vi "SEQ Header Read.vi"(0 "refnum":refnum<file>, 11 "error in":errorcluster) -> (4 "refnum out":refnum<file>, 6 "# of Frames":i16, 8 "AOI List":i16[][](array[numeric]), 10 "Header Info":T1, 15 "error out":errorcluster)   [LabVIEW 2011]
panel:
  # "Reading Sequence File Header"
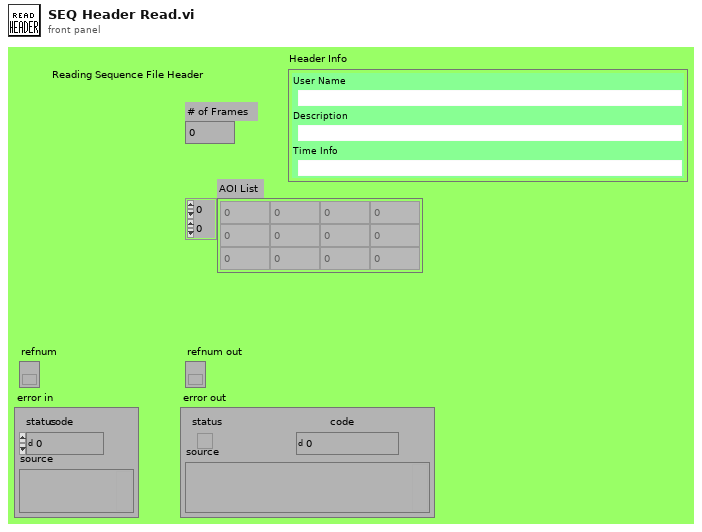
[diagram p1: front panel]
types:
  T1 = cluster{"User Name":string, "Description":string, "Time Info":string}
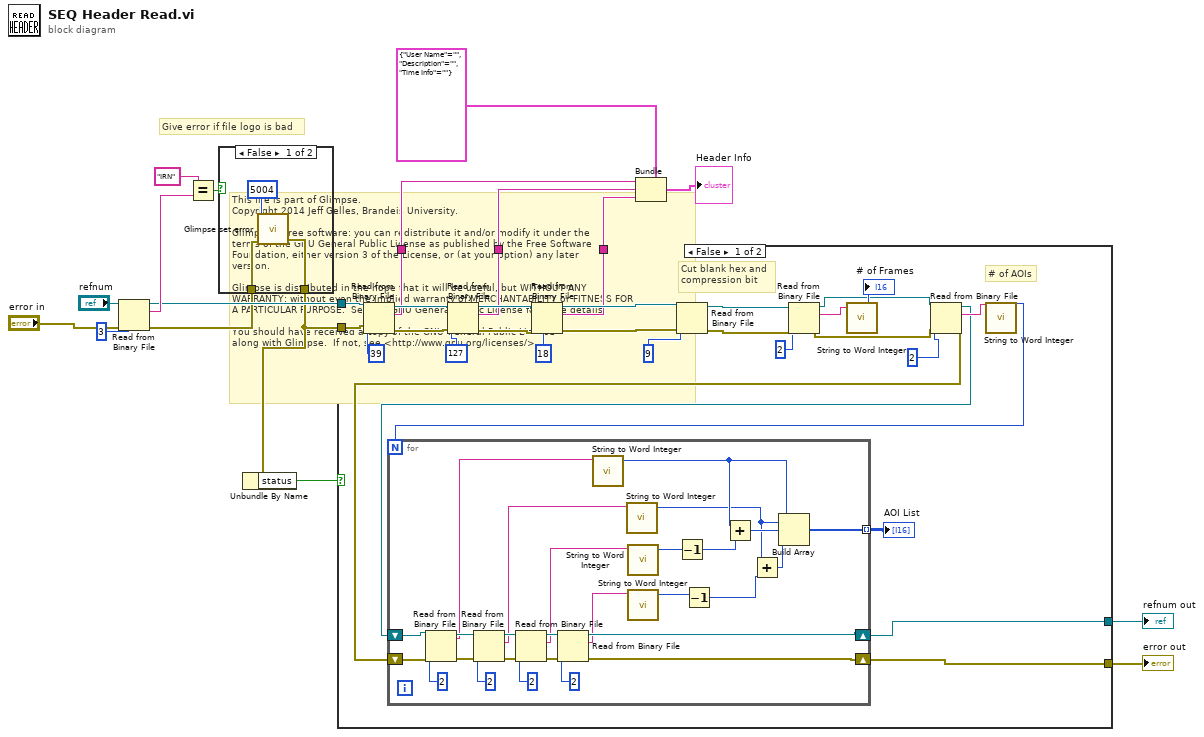
[diagram p0: block diagram]
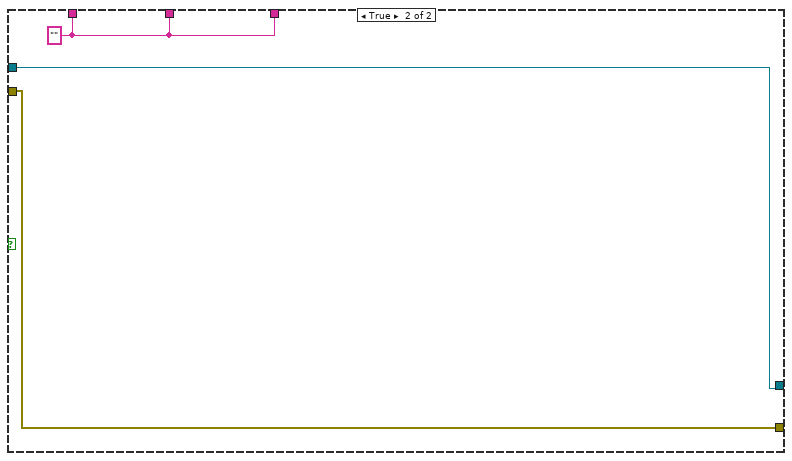
[diagram p2: hidden frame]
diagram:
  # "This file is part of Glimpse. \nCopyright 2014 Jeff Gelles, Brandeis University.    \n\nGlimpse is free software: you can redistribute it and/or modify it under the \nterms of the GNU General Public License as published by the Free Software \nFoundation, either version 3 of the License, or (at your option) any later \nversion.\n\nGlimpse is distributed in the hope that it will be useful, but WITHOUT ANY \nWARRANTY; without even the implied warranty of MERCHANTABILITY or FITNESS FOR \nA PARTICULAR PURPOSE.  See the GNU General Public License for more details.\n\nYou should have received a copy of the GNU General Public License\nalong with Glimpse.  If not, see <http://www.gnu.org/licenses/>."
  # "Give error if file logo is bad"
  n1 = Read from Binary File(8:"error in", 10:3 ("offset (0)"), 11:"refnum") -> (0:w10:errorcluster, 2:w13:string, 3:w12:refnum<file>)  [unwired: 4 out]
  n2 = Equal?(x="IRN" ("regular expression"), y=w13) -> (x = y?=w15:bool)
  n3 = case shown="False" w15 {
    tunnel: [w20 w21] -> w9
    tunnel: w10 -> [w19 w21]
    frame False {
      (unwired) FALSE
      n4 = call "Glimpse set error.vi"("code"=5004, "error in"=w19) -> ("error out"=w20:errorcluster)  [unwired: 1 in, 5 out]
    }
    frame True {
    }
  }
  n5 = Unbundle By Name(w9) -> ("status"=w8:bool)
  n6 = case shown="False" w8 {
    tunnel: w9 -> [w47 w80]
    tunnel: w12 -> [w46 w81]
    tunnel: [w26 w80] -> w7
    tunnel: [w25 w81] -> w6
    tunnel: [w24 w79] -> w5
    tunnel: [w23 w79] -> w4
    tunnel: [w22 w79] -> w2
    frame False {
      # "# of AOIs"
      # "Cut blank hex and\ncompression bit"
      n7 = Read from Binary File(8:w47, 10:39 ("offset (0)"), 11:w46) -> (0:w42:errorcluster, 2:w24:string, 3:w36:refnum<file>)  [unwired: 4 out]
      n8 = Read from Binary File(8:w42, 10:127 ("offset (0)"), 11:w36) -> (0:w41:errorcluster, 2:w23:string, 3:w35:refnum<file>)  [unwired: 4 out]
      n9 = Read from Binary File(8:w41, 10:18 ("offset (0)"), 11:w35) -> (0:w40:errorcluster, 2:w22:string, 3:w34:refnum<file>)  [unwired: 4 out]
      n10 = Read from Binary File(8:w40, 10:9 ("offset (0)"), 11:w34) -> (0:w39:errorcluster, 3:w33:refnum<file>)  [unwired: 5 out]
      n11 = Read from Binary File(8:w39, 10:2 ("offset (0)"), 11:w33) -> (0:w38:errorcluster, 2:w32:string, 3:w37:refnum<file>)  [unwired: 4 out]
      n12 = call "String to Word Integer.vi"("string"=w32) -> ("Integer"=→"# of Frames":i16)  [unwired: 5 out]
      n13 = Read from Binary File(8:w38, 10:2 ("offset (0)"), 11:w37) -> (0:w29:errorcluster, 2:w31:string, 3:w28:refnum<file>)  [unwired: 4 out]
      n14 = call "String to Word Integer.vi"("string"=w31) -> ("Integer"=w50:i16)  [unwired: 5 out]
      n15 = for {
        N: w50 -> [_]
        tunnel: [w73] -> w49 mode=indexing
        shift-right: [w59] -> w25
        shift-left: w28 -> [w61]
        shift-right: [w60] -> w26
        shift-left: w29 -> [w62]
        n16 = Read from Binary File(8:w62, 10:2 ("offset (0)"), 11:w61) -> (0:w70:errorcluster, 2:w55:string, 3:w69:refnum<file>)  [unwired: 4 out]
        n17 = Read from Binary File(8:w70, 10:2 ("offset (0)"), 11:w69) -> (0:w67:errorcluster, 2:w56:string, 3:w66:refnum<file>)  [unwired: 4 out]
        n18 = Read from Binary File(8:w67, 10:2 ("offset (0)"), 11:w66) -> (0:w64:errorcluster, 2:w57:string, 3:w63:refnum<file>)  [unwired: 4 out]
        n19 = Read from Binary File(8:w64, 10:2 ("offset (0)"), 11:w63) -> (0:w60:errorcluster, 2:w58:string, 3:w59:refnum<file>)  [unwired: 4 out]
        n20 = call "String to Word Integer.vi"("string"=w55) -> ("Integer"=w78:i16)  [unwired: 5 out]
        n21 = call "String to Word Integer.vi"("string"=w56) -> ("Integer"=w74:i16)  [unwired: 5 out]
        n22 = call "String to Word Integer.vi"("string"=w57) -> ("Integer"=w77:i16)  [unwired: 5 out]
        n23 = call "String to Word Integer.vi"("string"=w58) -> ("Integer"=w53:i16)  [unwired: 5 out]
        n24 = Decrement(x=w77) -> (x-1=w54:i16)
        n25 = Decrement(x=w53) -> (x-1=w52:i16)
        n26 = Add(x=w78, y=w54) -> (x+y=w76:i16)
        n27 = Add(x=w74, y=w52) -> (x+y=w75:i16)
        n28 = Build Array(w78, w74, w76, w75) -> (w73:i16[])
      }
      "AOI List" <- w49
    }
    frame True {
      w79 = "" ("User Name")
    }
  }
  "error out" <- w7
  "refnum out" <- w6
  n29 = Bundle(cluster=T1 {"User Name"="", "Description"="", "Time Info"=""} ("Header Info 2"), "User Name"=w5, "Description"=w4, "Time Info"=w2) -> (→"Header Info":T1)
